vi "DSF.Engine.Plugin.Set Timing.vi"(10 "Timing":refnum<class "Engine Timing.lvclass">, 11 "Plugin in":refnum<class "DSF.Engine.Plugin.lvclass">) -> (3 "Plugin out":refnum<class "DSF.Engine.Plugin.lvclass">)   [LabVIEW 2017, in "Data Sharing Framework Engine.lvlib" / "DSF.Engine.Plugin.lvclass"]
uses:
  DSF.Engine.Plugin.lvclass
  Source/Data Sharing Framework Core/Engine/Timing/Engine Timing.lvclass
  DSF.Engine.Plugin.lvclass/DSF.Engine.Plugin.ctl
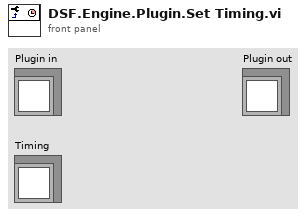
[diagram p1: front panel]
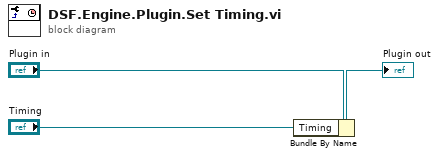
[diagram p0: block diagram]
diagram:
  n1 = Bundle By Name(cluster="Plugin in", "Timing"="Timing") -> (→"Plugin out":refnum<class "DSF.Engine.Plugin.lvclass">)
